vi "Core Action.vi"(8 "error in (no error)":errorcluster, 10 "SECS-II Class":refnum<class "SECS-II Class.lvclass">, 11 "Host Requests Current Status Variable Value in":refnum<class "03-Host Requests Current Status Variable Value.lvclass">) -> (0 "error out":errorcluster, 2 "SECS-II Class Out":refnum<class "SECS-II Class.lvclass">, 3 "Host Requests Current Status Variable Value out":refnum<class "03-Host Requests Current Status Variable Value.lvclass">)   [LabVIEW 2020, in "SECS Scenarios.lvlib" / "03-Host Requests Current Status Variable Value.lvclass"]
uses:
  03-Host Requests Current Status Variable Value.lvclass
  D:/Dropbox/SECS/SECS_GEM v1.1.0/Com/SECS Scenarios/Scenarios Class/Scenarios Class.lvclass
  SECS Communication/SECS-II Class/SECS-II Class.lvclass
  SECS Communication/S1 Message Class/S1 Message Class.lvclass
  D:/Dropbox/SECS/SECS_GEM v1.1.0/Com/SECS Communication/SECS-II Class/SECS-II Class.lvclass
  Scenarios Class/Scenarios Class.lvclass/Scenarios Class.ctl
  Scenarios Class/Reply State.ctl
  SECS Communication/SECS-II Class/Format Code.ctl
  Scenarios Class/Write Reply State.vi
  Scenarios Class/Read HSMS Class.vi
  SECS Communication/SECS Data Class/Get SVID Data.vi
  SECS Communication/SECS Data Class/Get All SVID Data.vi
  SECS Communication/HSMS Class/HSMS Class.lvclass
  SECS Communication/SECS Data Class/SECS Data Class.lvclass
  Scenarios Class/Scenarios Class.lvclass
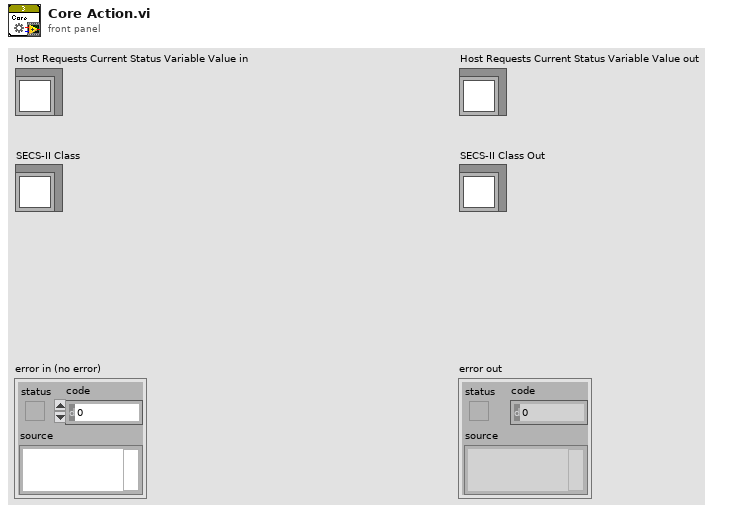
[diagram p1: front panel]
types:
  T1 = typedef "SECS Scenarios.lvlib/Scenarios Class.lvclass/Reply State.ctl" = enum16{"OK", "Illegal Data", "Unknown Stream", "Unknown Function", "Off-Line", "T3 Timeout", "Inner-Timeout"}
  T2 = typedef "SECS Communication.lvlib/SECS-II Class.lvclass/Format Code.ctl" = enum16{"L", "A", "B", "Boolean", "J", "I1", "I2", "I4", "I8", "U1", "U2", "U4", "U8", "F4", "F8", "Char"}
  T3 = typedef "SECS Communication.lvlib/SECS Data Class.lvclass/SVID Data.ctl" = cluster{"SVID":u32, "Name":string, "Description":string, "Format Code":T2, "Unit":string, "Source":string, "Data":variant}
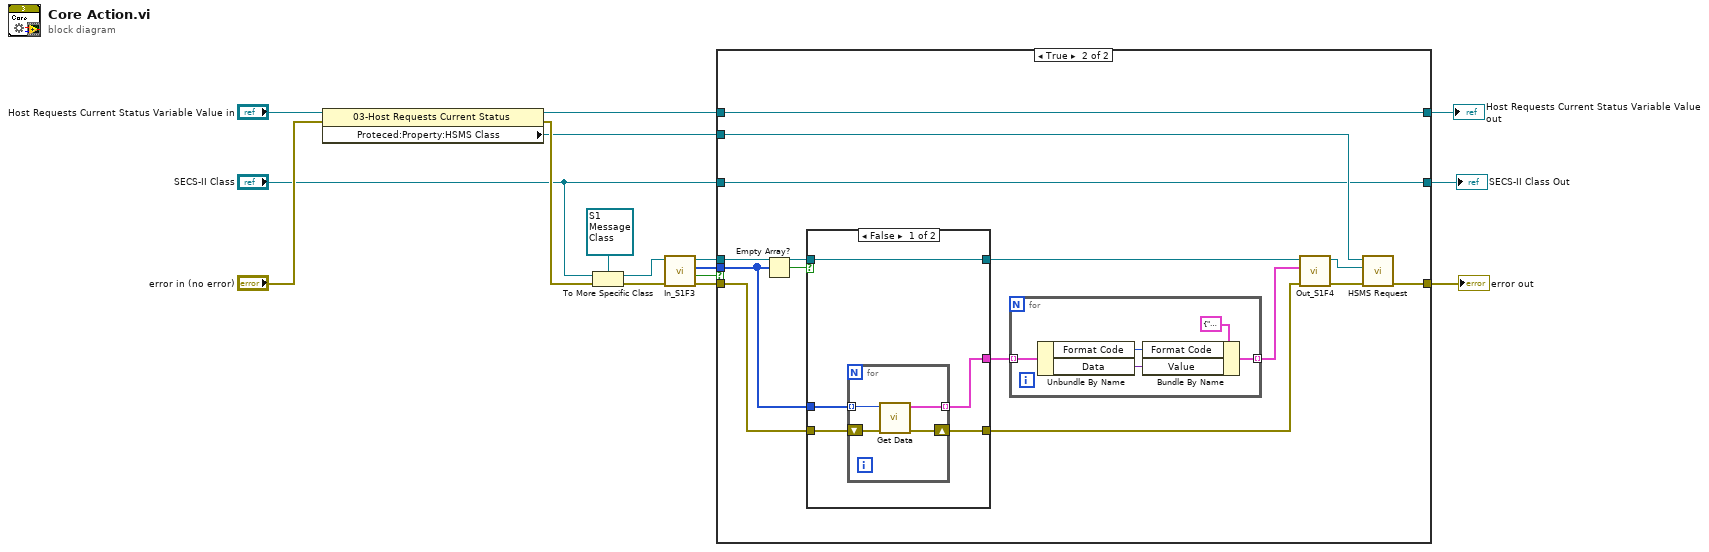
[diagram p0: block diagram]
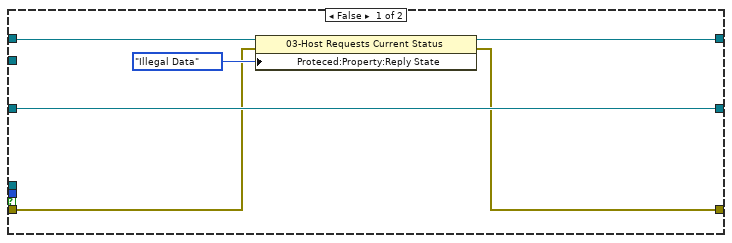
[diagram p2: hidden frame]
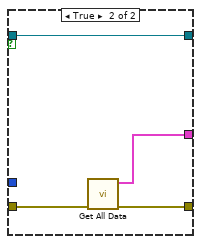
[diagram p3: hidden frame]
diagram:
  n1 = property class="03-Host Requests Current Status"(reference="Host Requests Current Status Variable Value in", error in="error in (no error)") -> (reference out=w2:refnum<class "03-Host Requests Current Status Variable Value.lvclass">, error out=w15:errorcluster, "Proteced:Property:HSMS Class"=w12:refnum<class "HSMS Class.lvclass">)
  n2 = To More Specific Class(target class=refnum<class "S1 Message Class.lvclass"> refnum ("S1 Message Class in"), reference="SECS-II Class", error in=w15) -> (specific class reference=w13:refnum<class "S1 Message Class.lvclass">, error out=w14:errorcluster)
  n3 = call "In_S1F3.vi"("error in (no error)"=w14, "S1 Message Class in"=w13) -> ("error out"=w7:errorcluster, "OK?"=w5:bool, "Status Variable ID(SVID)"=w6:u32[], "S1 Message Class out"=w8:refnum<class "S1 Message Class.lvclass">)  [unwired: 6 in]
  n4 = case shown="True" w5 {
    tunnel: w12 -> [_ w34]
    tunnel: [w17 w32] -> w9
    tunnel: w8 -> [_ w31]
    tunnel: w7 -> [w18 w28]
    tunnel: w6 -> [_ w27]
    tunnel: [w20 w24] -> w4
    tunnel: "SECS-II Class" -> [w20 w24]
    tunnel: w2 -> [w22 w23]
    tunnel: [w21 w23] -> w1
    frame False {
      n5 = property class="03-Host Requests Current Status"(reference=w22, error in=w18, "Proteced:Property:Reply State"=Reply_State."Illegal Data" ("Reply State")) -> (reference out=w21:refnum<class "03-Host Requests Current Status Variable Value.lvclass">, error out=w17:errorcluster)
    }
    frame True {
      n6 = Empty Array?(array=w27) -> (empty?=w26:bool)
      n7 = case shown="False" w26 {
        tunnel: w28 -> [w41 w49]
        tunnel: [w40 w47] -> w29
        tunnel: [w39 w48] -> w25
        tunnel: w27 -> [w38 _]
        tunnel: w31 -> [w37 w46]
        tunnel: [w37 w46] -> w30
        frame False {
          n8 = for {
            tunnel: w38 -> [w44] mode=indexing
            shift-right: [w43] -> w39
            shift-left: w41 -> [w45]
            tunnel: [w42] -> w40 mode=indexing
            n9 = call-poly "Get Data.vi"("error in"=w45, "SVID"=w44) -> ("error out"=w43:errorcluster, "SVID Data"=w42:T3)  [unwired: 7 in, 1 out]
          }
        }
        frame True {
          n10 = call-poly "Get All Data.vi"("error in (no error)"=w49) -> ("error out"=w48:errorcluster, "SVID Data"=w47:T3[])  [unwired: 9 in]
        }
      }
      n11 = for {
        tunnel: [w53] -> w33 mode=indexing
        tunnel: w29 -> [w50] mode=indexing
        n12 = Unbundle By Name(w50) -> ("Format Code"=w54:T2, "Data"=w51:variant)
        n13 = Bundle By Name(cluster=cluster{"Format Code":T2, "Value":variant} {"Format Code"=enum."A", "Value"=variant} ("SV"), "Format Code"=w54, "Value"=w51) -> (w53:cluster{"Format Code":T2, "Value":variant})
      }
      n14 = call "Out_S1F4.vi"("error in (no error)"=w25, "SV"=w33, "S1 Message Class in"=w30) -> ("error out"=w36:errorcluster, "S1 Message Class out"=w35:refnum<class "S1 Message Class.lvclass">)  [unwired: 7 in]
      n15 = call "HSMS Request.vi"("error in (no error)"=w36, "SECS-II Class In"=w35, "HSMS Class in"=w34) -> ("error out"=w32:errorcluster)  [unwired: 7 in, 1 out]
    }
  }
  "error out" <- w9
  "Host Requests Current Status Variable Value out" <- w1
  "SECS-II Class Out" <- w4
